vi "Get Operator ID.vi"() -> (0 "Employee ID":string)   [LabVIEW 2013]
panel:
  in  "OK Button":bool
  in  "Enter Employee ID Number\n(4 digits)":string
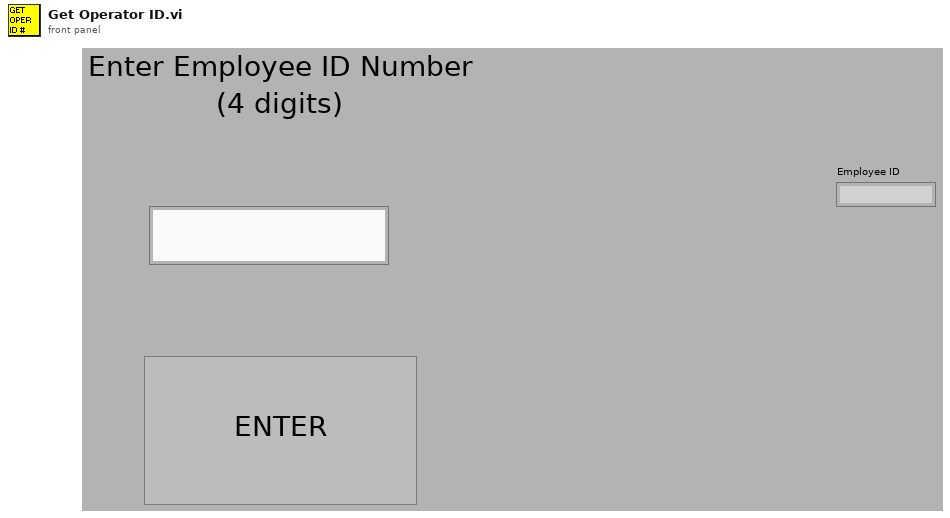
[diagram p1: front panel]
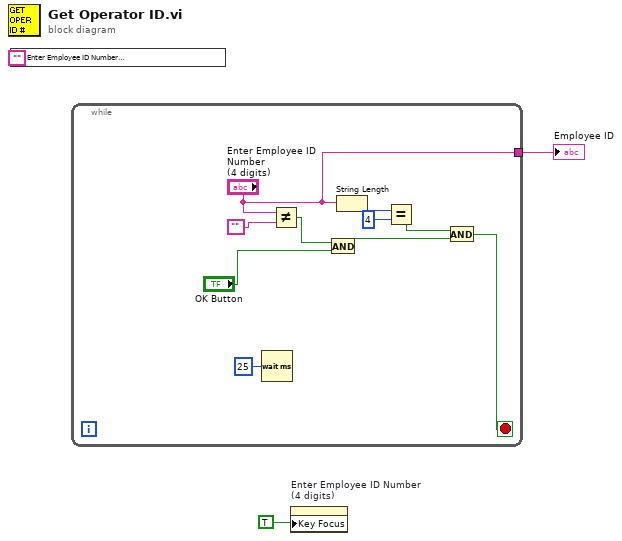
[diagram p0: block diagram]
diagram:
  n1 = local write "Enter Employee ID Number\n(4 digits)"("") -> ()
  n2 = while {
    tunnel: ["Enter Employee ID Number\n(4 digits)"] -> w1
    stop <- w5 stop-if-true
    n3 = Wait (ms)(milliseconds to wait=u32 25) -> ()  [unwired: 1 out]
    n4 = Not Equal?(x="Enter Employee ID Number\n(4 digits)", y="") -> (x != y?=w12:bool)
    n5 = And(x=w12, y="OK Button") -> (x .and. y?=w6:bool)
    n6 = String Length(string="Enter Employee ID Number\n(4 digits)") -> (length=w9:i32)
    n7 = Equal?(x=w9, y=4) -> (x = y?=w7:bool)
    n8 = And(x=w7, y=w6) -> (x .and. y?=w5:bool)
  }
  "Employee ID" <- w1
  n9 = property on="Enter Employee ID Number\n(4 digits)" class="Str"("Key Focus"=TRUE) -> ()  [unwired: 2 in, 2 out]
